vi "全局变量测试2.vi"() -> ()   [LabVIEW 2020]
panel:
  out "地址：":string
  out "电话：":string
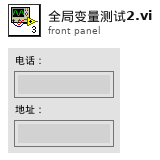
[diagram p1: front panel]
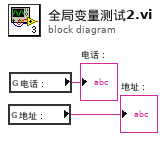
[diagram p0: block diagram]
diagram:
  n1 = global read "快捷购买信息.vi" "地址："() -> (→"地址：":string)
  n2 = global read "快捷购买信息.vi" "电话："() -> (→"电话：":string)
